vi "Create GUI element.vi"(8 "error in (no error)":errorcluster, 11 "Run Instance in":refnum<class "Run Instance.lvclass">) -> (0 "error out":errorcluster, 2 "Single RUN":T1, 3 "Run Instance out":refnum<class "Run Instance.lvclass">)   [LabVIEW 2020, in "Run Utilities.lvlib" / "Run Instance.lvclass"]
uses:
  Run Instance.lvclass
  Run Instance - GUI.ctl
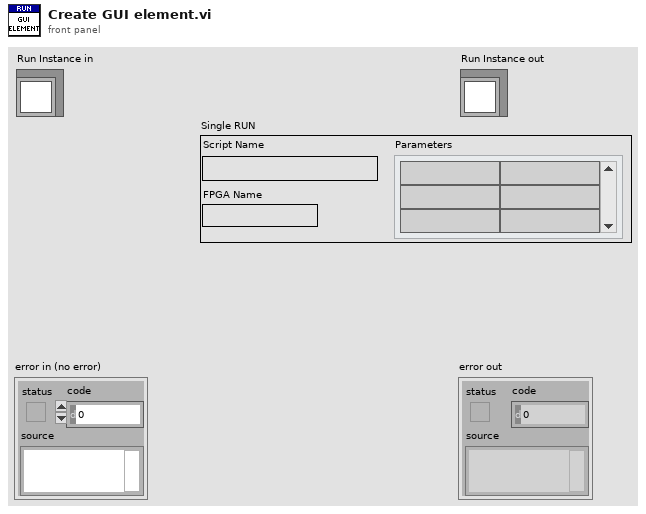
[diagram p1: front panel]
types:
  T1 = typedef "Run Utilities.lvlib/Run Instance.lvclass/Run Instance - GUI.ctl" = cluster{"Script Name":string, "Parameters":string[][], "FPGA Name":string}
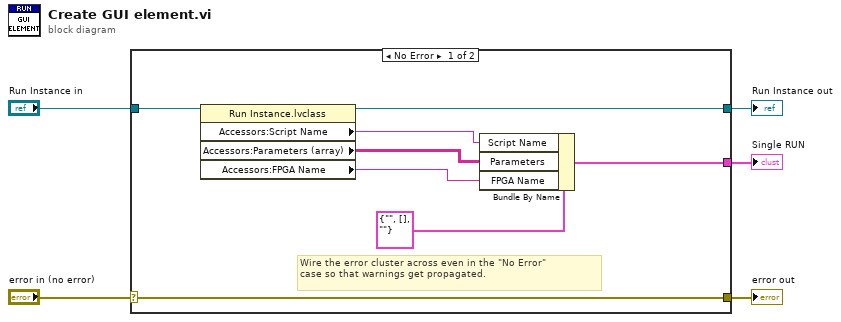
[diagram p0: block diagram]
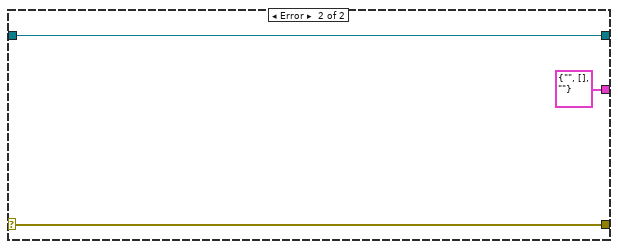
[diagram p2: hidden frame]
diagram:
  n1 = case shown="No Error" "error in (no error)" {
    selector: "error in (no error)" -> [w12 w16]
    tunnel: [w12 w16] -> w4
    tunnel: [w10 w15] -> w2
    tunnel: "Run Instance in" -> [w13 w15]
    tunnel: [w7 T1 {"Script Name"="", "Parameters"=[], "FPGA Name"=""} ("Single RUN")] -> w1
    frame No Error {
      # "Wire the error cluster across even in the \"No Error\"\ncase so that warnings get propagated."
      n2 = property class="Run Instance.lvclass"(reference=w13) -> (reference out=w10:refnum<class "Run Instance.lvclass">, "Accessors:Script Name"=w9:string, "Accessors:Parameters (array)"=w8:string[][], "Accessors:FPGA Name"=w6:string)  [unwired: 1 in, 1 out]
      n3 = Bundle By Name(cluster=T1 {"Script Name"="", "Parameters"=[], "FPGA Name"=""} ("Single RUN"), "Script Name"=w9, "Parameters"=w8, "FPGA Name"=w6) -> (w7:T1)
    }
    frame Error {
    }
  }
  "error out" <- w4
  "Run Instance out" <- w2
  "Single RUN" <- w1
